vi "Reshape Image x8 (SubVI).vi"(0 "Pixel Data In":u64, 5 "Pixel In Valid?":bool=TRUE, 10 "Block Size":u16=8, 12 "Image Width":u16=512) -> (14 "Pixel Data Out":u64, 19 "Pixel Out Valid?":bool)   [LabVIEW 2015]
uses:
  Controls (FPGA)/Image Block Readout.ctl
  Controls (FPGA)/Image Block Write.ctl
  <vilib>/rvi/DataTransferAndStorage/Container/Common/niFpgaContainerGetUniqueNameForEmu.vi
  <vilib>/rvi/DataTransferAndStorage/Container/Common/niFpgaContainerSetEmuInfo.vi
  <vilib>/rvi/eio/common/nirviEmuReportErrorAndStop.vi
  <vilib>/rvi/Memory/Memory_Emulation/nirvimemoryFastEmulation.vi
  <vilib>/rvi/Memory/Memory_Emulation/nirvimemoryEmulation.vi
  <vilib>/rvi/Emulation/niFpgaEmulationIsFPGAContextNoSignature.vi
  <vilib>/rvi/Emulation/niFpgaProcessEmulError.vi
  <vilib>/rvi/Emulation/niFpgaSctlEmulationGetInTimedLoop.vi
  <vilib>/rvi/errors/nirviReportUnexpectedCaseInternalError (U32).vi
  <vilib>/rvi/errors/niFpgaSetErrorForExecOnDevCompSimple.vi
  <vilib>/rvi/FIFO/Fifo_Resource/nirvififoEmulationSetSize.vi
  <vilib>/rvi/FIFO/Fifo_Resource/nirviFifoEmulationQueueMgr.vi
  <instcachedir>/0/nirviFifoEmulationQueueMgr_E5CAEC123FF24DC58D834DCA3CDAA9B5.lvgen/nirviFifoEmulationQueueMgr_E5CAEC123FF24DC58D834DCA3CDAA9B5_005.vi
  <vilib>/rvi/FIFO/Fifo_Resource/nirvififoEmulationDetermineInputValidOut.vi
  <vilib>/rvi/FIFO/Fifo_Resource/nirvififoEmulationCreateLock.vi
  <vilib>/rvi/FIFO/Fifo_Resource/nirvififoEmulationObtainLock.vi
  <vilib>/rvi/FIFO/Fifo_Resource/nirvififoEmulationReleaseLock.vi
  <vilib>/rvi/occurrence/nirviWaitOnOccurrenceBase.vi
  <vilib>/rvi/errors/nirviReportUnexpectedCaseInternalError.vi
  <vilib>/Utility/error.llb/Clear Errors.vi
  <vilib>/rvi/LocalResourceManager/LocalResourceManager.xnode
  <vilib>/rvi/DataTransferAndStorage/Container/XNode/niFpgaContainer.xnode
  <vilib>/rvi/FIFO/Fifo_Resource/nirvififoEmulationWrite.vi
  <vilib>/rvi/FIFO/Fifo_Resource/nirvififoEmulationRead.vi
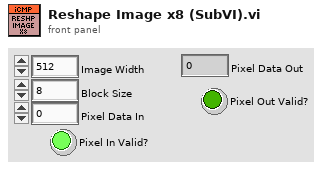
[diagram p1: front panel]
types:
  T1 = typedef "Image Block Readout.ctl" = enum16{"Sync Read", "Read Block Set 1", "Read Block Set 2"}
  T2 = typedef "Image Block Write.ctl" = enum16{"Block 1", "Block 2"}
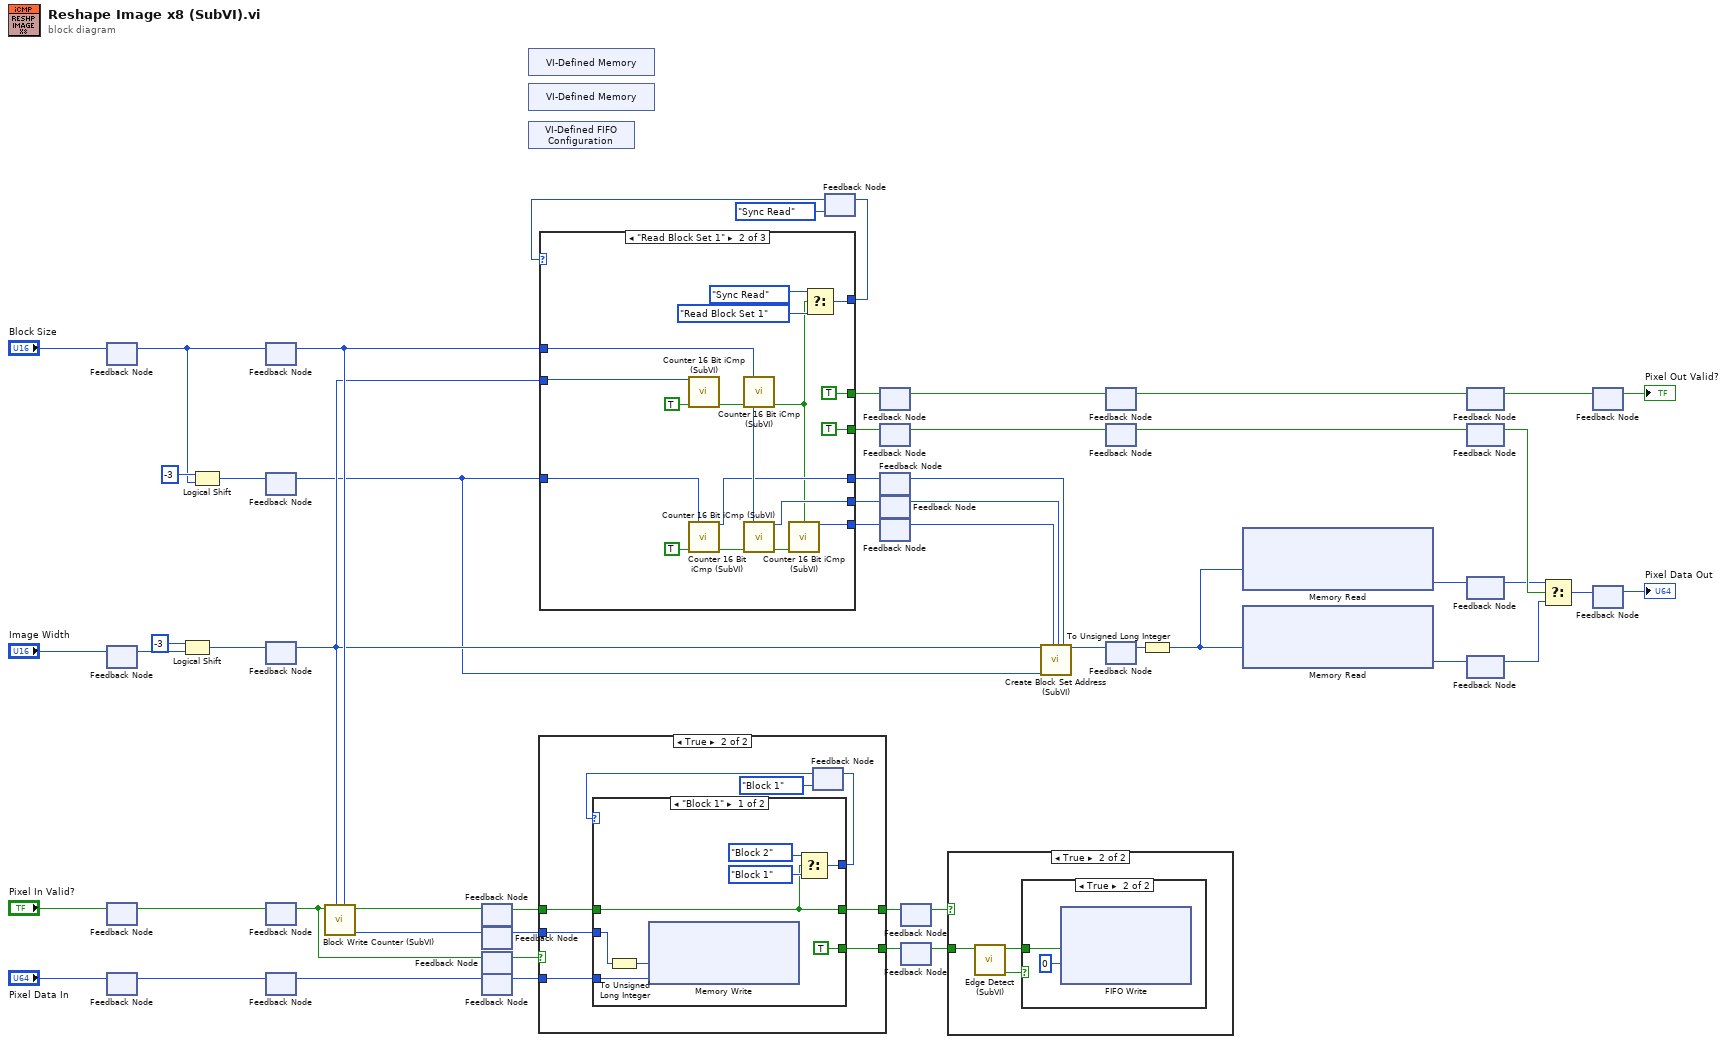
[diagram p0: block diagram]
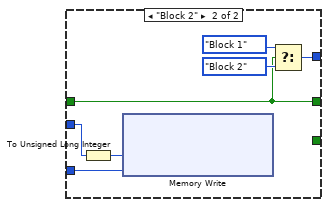
[diagram p5: hidden frame]
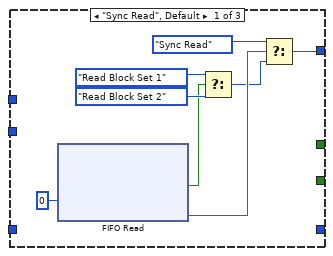
[diagram p6: hidden frame]
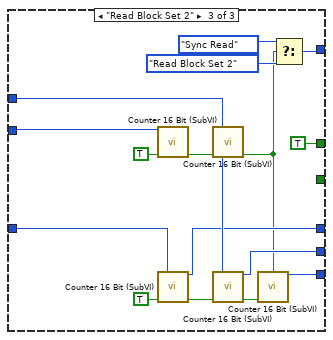
[diagram p7: hidden frame]
diagram:
  n1 = feedback-in #1("Block Size") -> ()
  n2 = feedback #1() -> (w7:u16)  [unwired: 1 in]
  n3 = feedback-in #2("Image Width") -> ()
  n4 = feedback #2() -> (w6:u16)  [unwired: 1 in]
  n5 = feedback-in #3("Pixel In Valid?") -> ()
  n6 = feedback #3() -> (w5:bool)  [unwired: 1 in]
  n7 = feedback-in #4("Pixel Data In") -> ()
  n8 = feedback #4() -> (w4:u64)  [unwired: 1 in]
  n9 = Logical Shift(y=i16 -3, x=w6) -> (x << y=w16:u16)
  n10 = Logical Shift(y=i16 -3, x=w7) -> (x << y=w12:u16)
  n11 = feedback-in #5(w7) -> ()
  n12 = feedback #5() -> (w11:u16)  [unwired: 1 in]
  n13 = feedback-in #6(w12) -> ()
  n14 = feedback #6() -> (w1:u16)  [unwired: 1 in]
  n15 = feedback-in #7(w16) -> ()
  n16 = feedback #7() -> (w10:u16)  [unwired: 1 in]
  n17 = feedback-in #8(w5) -> ()
  n18 = feedback #8() -> (w9:bool)  [unwired: 1 in]
  n19 = feedback-in #9(w4) -> ()
  n20 = feedback #9() -> (w8:u64)  [unwired: 1 in]
  n21 = call "Block Write Counter (SubVI).vi"("Block Size"=w11, "Image Width"=w10, "Pixel Valid?"=w9) -> ("Count"=w27:u16, "Count End?"=w28:bool)  [unwired: 7 in]
  n22 = feedback-in #10(w28) -> ()
  n23 = feedback #10() -> (w25:bool)  [unwired: 1 in]
  n24 = feedback-in #11(w27) -> ()
  n25 = feedback #11() -> (w24:u16)  [unwired: 1 in]
  n26 = feedback-in #12(w9) -> ()
  n27 = feedback #12() -> (w23:bool)  [unwired: 1 in]
  n28 = feedback-in #13(w8) -> ()
  n29 = feedback #13() -> (w22:u64)  [unwired: 1 in]
  n30 = xnode "VI-Defined Memory"() -> ()  [unwired: 1 out]
  n31 = xnode "VI-Defined Memory"() -> ()  [unwired: 1 out]
  n32 = xnode "VI-Defined FIFO Configuration"() -> ()  [unwired: 1 out]
  n33 = case shown="True" w23 {
    tunnel: w22 -> [_ w59]
    tunnel: w25 -> [_ w58]
    tunnel: w24 -> [_ w57]
    tunnel: [_ w56] -> w21
    tunnel: [_ w55] -> w20
    frame False {
    }
    frame True {
      n34 = feedback #14(Image_Block_Write."Block 1") -> (w61:T2)
      n35 = case shown="\"Block 1\"" w61 {
        tunnel: w57 -> [w70 w77]
        tunnel: w59 -> [w69 w76]
        tunnel: [w65 w72] -> w62
        tunnel: w58 -> [w63 w71]
        tunnel: [w63 w71] -> w56
        tunnel: [TRUE ("Enable") _] -> w55
        frame "Block 1" {
          n36 = To Unsigned Long Integer(number=w70) -> (unsigned 32bit integer=w68:u32)
          n37 = xnode ("Memory Write")("Address"=w68, "Data"=w69) -> ()  [unwired: 1 in, 1 out]
          n38 = Select(t=Image_Block_Write."Block 2", s=w63, f=Image_Block_Write."Block 1") -> (s? t:f=w65:T2)
        }
        frame "Block 2" {
          n39 = To Unsigned Long Integer(number=w77) -> (unsigned 32bit integer=w75:u32)
          n40 = xnode ("Memory Write")("Address"=w75, "Data"=w76) -> ()  [unwired: 1 in, 1 out]
          n41 = Select(t=Image_Block_Write."Block 1", s=w71, f=Image_Block_Write."Block 2") -> (s? t:f=w72:T2)
        }
      }
      n42 = feedback-in #14(w62) -> ()
    }
  }
  n43 = feedback #15(Image_Block_Readout."Sync Read") -> (w31:T1)
  n44 = case shown="\"Read Block Set 1\"" w31 {
    tunnel: [w84 w99 w115] -> w30
    tunnel: w11 -> [_ w95 w111]
    tunnel: [_ w93 w109] -> w35
    tunnel: [_ w92 w108] -> w36
    tunnel: [_ w91 w107] -> w37
    tunnel: [_ TRUE ("Auto RESET") _] -> w34
    tunnel: [_ TRUE ("Auto RESET") TRUE ("Auto RESET")] -> w33
    tunnel: w10 -> [_ w87 w104]
    tunnel: w1 -> [_ w86 w103]
    frame "Sync Read", Default {
      n45 = xnode ("FIFO Read")("Timeout"=0) -> ("Element"=w79:bool, "Timed Out?"=w82:bool)  [unwired: 1 in, 1 out]
      n46 = Select(t=Image_Block_Readout."Read Block Set 1", s=w79, f=Image_Block_Readout."Read Block Set 2") -> (s? t:f=w78:T1)
      n47 = Select(t=Image_Block_Readout."Sync Read", s=w82, f=w78) -> (s? t:f=w84:T1)
    }
    frame "Read Block Set 1" {
      n48 = call "Counter 16 Bit iCmp (SubVI).vi"("Max. Count"=w87, "Enable"=TRUE) -> ("Count End?"=w94:bool)  [unwired: 11 in, 2 out]
      n49 = call "Counter 16 Bit iCmp (SubVI).vi"("Max. Count"=w86, "Enable"=TRUE) -> ("Count"=w93:u16, "Count End?"=w97:bool)  [unwired: 11 in, 1 out]
      n50 = call "Counter 16 Bit iCmp (SubVI).vi"("Max. Count"=w95, "Enable"=w94) -> ("Count End?"=w88:bool)  [unwired: 11 in, 2 out]
      n51 = call "Counter 16 Bit iCmp (SubVI).vi"("Max. Count"=w95, "Enable"=w97) -> ("Count"=w92:u16, "Count End?"=w96:bool)  [unwired: 11 in, 1 out]
      n52 = call "Counter 16 Bit iCmp (SubVI).vi"("RESET"=w88, "Enable"=w96) -> ("Count"=w91:u16)  [unwired: 11 in, 2 out]
      n53 = Select(t=Image_Block_Readout."Sync Read", s=w88, f=Image_Block_Readout."Read Block Set 1") -> (s? t:f=w99:T1)
    }
    frame "Read Block Set 2" {
      n54 = call "Counter 16 Bit (SubVI).vi"("Max. Count"=w104, "Enable"=TRUE) -> ("Count End?"=w110:bool)  [unwired: 11 in, 2 out]
      n55 = call "Counter 16 Bit (SubVI).vi"("Max. Count"=w103, "Enable"=TRUE) -> ("Count"=w109:u16, "Count End?"=w113:bool)  [unwired: 11 in, 1 out]
      n56 = call "Counter 16 Bit (SubVI).vi"("Max. Count"=w111, "Enable"=w110) -> ("Count End?"=w105:bool)  [unwired: 11 in, 2 out]
      n57 = call "Counter 16 Bit (SubVI).vi"("Max. Count"=w111, "Enable"=w113) -> ("Count"=w108:u16, "Count End?"=w112:bool)  [unwired: 11 in, 1 out]
      n58 = call "Counter 16 Bit (SubVI).vi"("RESET"=w105, "Enable"=w112) -> ("Count"=w107:u16)  [unwired: 11 in, 2 out]
      n59 = Select(t=Image_Block_Readout."Sync Read", s=w105, f=Image_Block_Readout."Read Block Set 2") -> (s? t:f=w115:T1)
    }
  }
  n60 = feedback-in #15(w30) -> ()
  n61 = feedback #16() -> (w42:bool)  [unwired: 1 in]
  n62 = feedback-in #16(w33) -> ()
  n63 = feedback #17() -> (w43:bool)  [unwired: 1 in]
  n64 = feedback-in #17(w34) -> ()
  n65 = feedback #18() -> (w38:u16)  [unwired: 1 in]
  n66 = feedback-in #18(w35) -> ()
  n67 = feedback #19() -> (w39:u16)  [unwired: 1 in]
  n68 = feedback-in #19(w36) -> ()
  n69 = feedback #20() -> (w40:u16)  [unwired: 1 in]
  n70 = feedback-in #20(w37) -> ()
  n71 = feedback-in #21(w21) -> ()
  n72 = feedback #21() -> (w19:bool)  [unwired: 1 in]
  n73 = feedback-in #22(w20) -> ()
  n74 = feedback #22() -> (w18:bool)  [unwired: 1 in]
  n75 = case shown="True" w19 {
    tunnel: w18 -> [_ w119]
    frame False {
    }
    frame True {
      n76 = call "Edge Detect (SubVI).vi"("TTL In"=w119) -> ("Edge?"=w121:bool, "Rising Edge"=w120:bool)  [unwired: 8 in, 1 out]
      n77 = case shown="True" w121 {
        tunnel: w120 -> [_ w122]
        frame False {
        }
        frame True {
          n78 = xnode ("FIFO Write")("Element"=w122, "Timeout"=0) -> ()  [unwired: 1 in, 2 out]
        }
      }
    }
  }
  n79 = call "Create Block Set Address (SubVI).vi"("Image Width"=w10, "Block Size"=w1, "Block N"=w40, "Block Y"=w39, "Block X"=w38) -> ("Address"=w41:u16)  [unwired: 14 in]
  n80 = feedback #23() -> (w48:bool)  [unwired: 1 in]
  n81 = feedback-in #23(w42) -> ()
  n82 = feedback #24() -> (w49:bool)  [unwired: 1 in]
  n83 = feedback-in #24(w43) -> ()
  n84 = feedback #25() -> (w44:u16)  [unwired: 1 in]
  n85 = feedback-in #25(w41) -> ()
  n86 = To Unsigned Long Integer(number=w44) -> (unsigned 32bit integer=w45:u32)
  n87 = xnode ("Memory Read")("Address"=w45) -> ("Data"=w47:u64)  [unwired: 1 in, 1 out]
  n88 = xnode ("Memory Read")("Address"=w45) -> ("Data"=w46:u64)  [unwired: 1 in, 1 out]
  n89 = feedback #26() -> (w50:bool)  [unwired: 1 in]
  n90 = feedback-in #26(w48) -> ()
  n91 = feedback #27() -> (w53:bool)  [unwired: 1 in]
  n92 = feedback-in #27(w49) -> ()
  n93 = feedback #28() -> (w51:u64)  [unwired: 1 in]
  n94 = feedback-in #28(w47) -> ()
  n95 = feedback #29() -> (w52:u64)  [unwired: 1 in]
  n96 = feedback-in #29(w46) -> ()
  n97 = Select(t=w51, s=w53, f=w52) -> (s? t:f=w54:u64)
  n98 = feedback-in #30(w50) -> ()
  n99 = feedback #30() -> (→"Pixel Out Valid?":bool)  [unwired: 1 in]
  n100 = feedback-in #31(w54) -> ()
  n101 = feedback #31() -> (→"Pixel Data Out":u64)  [unwired: 1 in]
